vi "HumanGlobal.vi"() -> ()   [LabVIEW 2023]
panel:
  out "AutoSpeakerAngleEnabled":bool
  out "InsideWing":bool
  out "InRange":bool
  out "OnTargetSpeaker":bool
  out "DesiredAngularSpeed (degree/s)":dbl
  out "DesiredAngleToSpeaker (degrees)":dbl
  out "DistanceToSpeaker (m)":dbl
  out "CurrentAction":string
  out "Reverse":bool
  out "StateChange":bool
  out "DPadLeft":bool
  out "DPadRight":bool
  out "DPadDown":bool
  out "DPadUp":bool
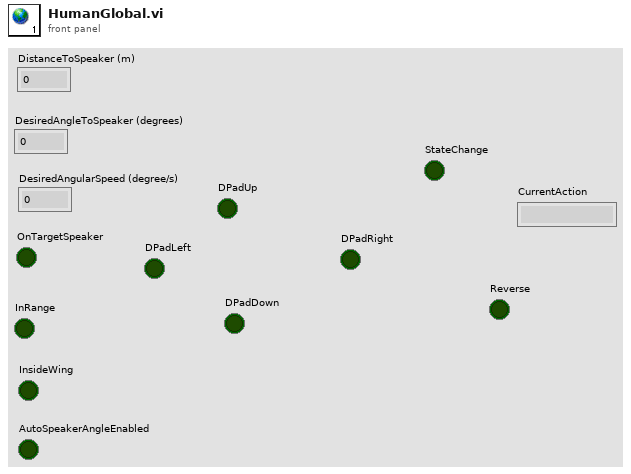
[diagram p1: front panel]
diagram:
